vi "Get Window RefNum Wrapper.vi"(8 "error in (no error)":T1, 11 "Window Name":string) -> (0 "error out":errorcluster, 3 "window refnum":T2)   [LabVIEW 2020, in "MacroAssert.lvlib"]
doc: "Wrapper around \"Get Window RefNum.vi\" that checks <B>Window Name</B> for certain program-defined strings to get specific windows without knowing what the window name is."
uses:
  MacroAssert.lvlib
  SubVIs/Win Util/Window Refnum.ctl
  SubVIs/Win Util/Win Util.lvlib
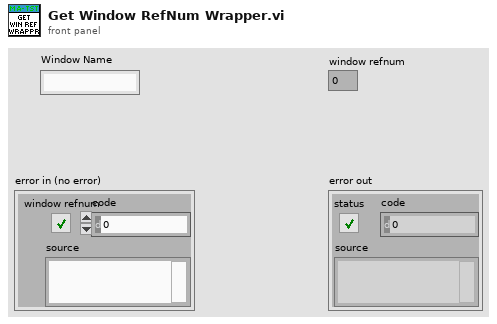
[diagram p1: front panel]
types:
  T1 = cluster{"window refnum":bool, "code":i32, "source":string}
  T2 = typedef "MacroAssert.lvlib/Win Util.lvlib/Window Refnum.ctl" = u64
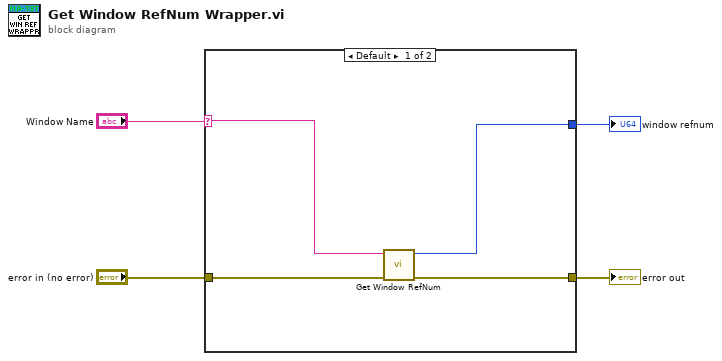
[diagram p0: block diagram]
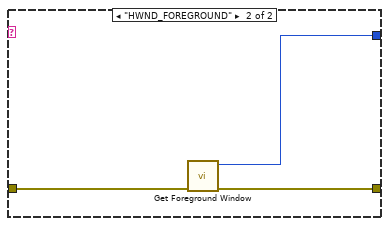
[diagram p2: hidden frame]
diagram:
  n1 = case shown="Default" "Window Name" {
    selector: "Window Name" -> [w7 _]
    tunnel: "error in (no error)" -> [w8 w11]
    tunnel: [w6 w10] -> w2
    tunnel: [w5 w9] -> w1
    frame Default {
      n2 = call "Get Window RefNum.vi"("error in"=w8, "window name (\"\")"=w7) -> ("error out"=w6:errorcluster, "window refnum (NaWR)"=w5:T2)  [unwired: 6 in]
    }
    frame "HWND_FOREGROUND" {
      n3 = call "Get Foreground Window.vi"("error in"=w11) -> ("error out"=w10:errorcluster, "window refnum out"=w9:T2)  [unwired: 8 in, 1 out]
    }
  }
  "window refnum" <- w1
  "error out" <- w2
